vi "variables offset.vi"() -> ()   [LabVIEW 2015]
panel:
  out "valor 8":dbl
  out "valor 7":dbl
  out "valor 6":dbl
  out "valor 5":dbl
  out "valor 4":dbl
  out "valor 3":dbl
  out "valor 2":dbl
  out "valor 1":dbl
  out "tensiometro":bool
  out "presion":bool
  out "carga":bool
  out "lvdt":bool
  out "galga 4":bool
  out "galga 3":bool
  out "galga 2":bool
  out "galga 1":bool
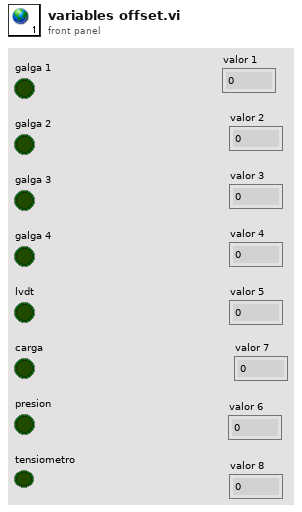
[diagram p1: front panel]
diagram:
